vi "RFSG Config - PAE.vi"(8 "error in":errorcluster, 10 "RFSG Settings":T2 {"Attenuation"."s2p File"."RFSG S-parameters Orientation" items=["Port1 Towards DUT"=24000, "Port2 Towards DUT"=24001]; "Attenuation"."Contant Attenuation"."RFSG External Attenuation (dB)" format="%.2f"}, 11 "PAE Reference in":T1) -> (0 "error out":errorcluster, 3 "PAE Reference out":T1)   [LabVIEW 2023]
uses:
  <vilib>/niPAEML/Typedefs/Session Handle.ctl
  <vilib>/niPAEML/PAE Reference.lvclass
  Controls/RFSG Config - Compression.ctl
  FPT Shared VIs/De-embedding/RFsg Config.ctl
  <vilib>/niPAEML/PAE Measurement.lvlib
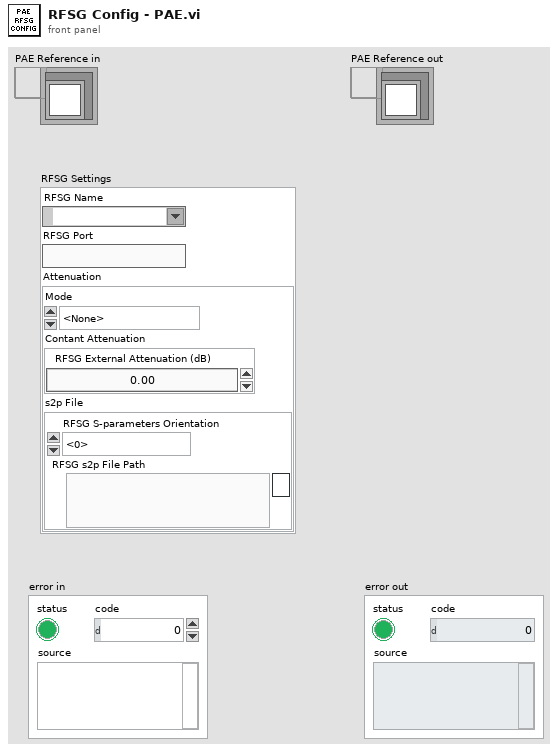
[diagram p1: front panel]
types:
  T1 = typedef "PAE Measurement.lvlib/PAE Reference.lvclass/Session Handle.ctl" = refnum<data-value>
  T2 = typedef "RFSG Config - Compression.ctl" = cluster{"RFSG Name":refnum<k15>, "RFSG Port":string, "Attenuation":cluster{"Mode":enum32{"<None>", "Constant Attenuation", "s2p File"}, "Contant Attenuation":cluster{"RFSG External Attenuation (dB)":dbl}, "s2p File":cluster{"RFSG S-parameters Orientation":i32, "RFSG s2p File Path":path}}}
  T3 = typedef "RFsg Config.ctl" = cluster{"RFSG Name":refnum<k15>, "RFSG Port":string, "Attenuation":cluster{"Mode":enum32{"<None>", "Constant Attenuation", "s2p File"}, "Contant Attenuation":cluster{"RFSG External Attenuation (dB)":dbl}, "s2p File":cluster{"RFSG S-parameters Orientation":i32, "RFSG Attenuation s2p Path Name":string, "RFSG s2p File Path":path}}}
  T4 = enum32{"<None>", "Constant Attenuation", "s2p File"}
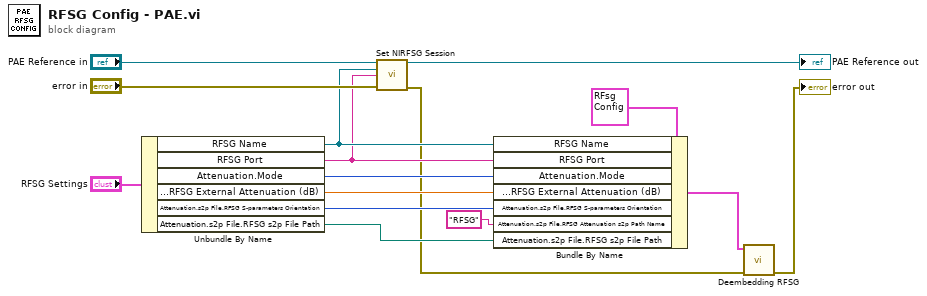
[diagram p0: block diagram]
diagram:
  n1 = Unbundle By Name("RFSG Settings") -> ("RFSG Name"=w9:refnum<k15>, "RFSG Port"=w8:string, "Attenuation.Mode"=w7:T4, "Attenuation.Contant Attenuation.RFSG External Attenuation (dB)"=w6:dbl, "Attenuation.s2p File.RFSG S-parameters Orientation"=w5:i32, "Attenuation.s2p File.RFSG s2p File Path"=w3:path)
  n2 = call <vilib>:"Set NIRFSG Session.vi"("PAE Reference In"="PAE Reference in", "NI RFSG Instrument Handle"=w9, "NI RFSG Port"=w8, "error in"="error in") -> ("PAE Reference Out"=→"PAE Reference out":T1, "error out"=w2:errorcluster)  [unwired: 10 in]
  n3 = Bundle By Name(cluster=T3 {"RFSG Name"="5842_0", "RFSG Port"="", "Attenuation"={"Mode"=enum."Constant Attenuation", "Contant Attenuation"={"RFSG External Attenuation (dB)"=2.0}, "s2p File"={"RFSG S-parameters Orientation"=24000, "RFSG Attenuation s2p Path Name"="", "RFSG s2p File Path"=path ""}}} ("RFSG Settings"), "RFSG Name"=w9, "RFSG Port"=w8, "Attenuation.Mode"=w7, "Attenuation.Contant Attenuation.RFSG External Attenuation (dB)"=w6, "Attenuation.s2p File.RFSG S-parameters Orientation"=w5, "Attenuation.s2p File.RFSG Attenuation s2p Path Name"="RFSG" ("RFSG Attenuation Path Name"), "Attenuation.s2p File.RFSG s2p File Path"=w3) -> (w11:T3)
  n4 = call "Deembedding RFSG.vi"("error in"=w2, "RFSG Settings"=w11) -> ("error out"=→"error out":errorcluster)  [unwired: 8 in, 1 out]
